vi "Temporarily Grant File Permissions.vi"(8 "error in":errorcluster) -> (0 "error out":errorcluster)   [LabVIEW 2015]
panel:
  out "permissions":i16
  out "path out":path
  in  "others":T1={"read"=TRUE, "write"=TRUE, "execute"=TRUE}
  in  "group":T1={"read"=TRUE, "write"=TRUE, "execute"=TRUE}
  in  "user":T1={"read"=TRUE, "write"=TRUE, "execute"=TRUE}
  in  "path":path=path "C:/Program Files (x86)/National Instruments/RT Images/User Components"
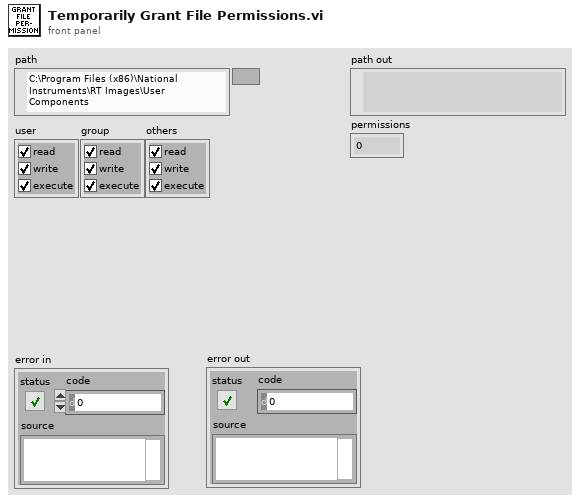
[diagram p1: front panel]
types:
  T1 = cluster{"read":bool, "write":bool, "execute":bool}
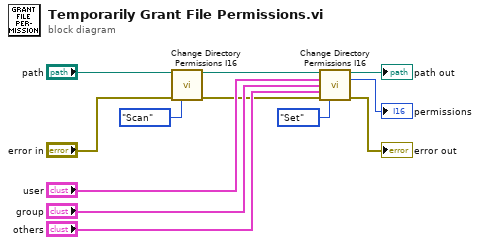
[diagram p0: block diagram]
diagram:
  n1 = call "Change Directory Permissions I16.vi"("path"="path", "error in"="error in", "Action (Get)"=enum16{"Get", "Scan", "Set", "Restore"}."Scan") -> ("path out"=w2:path, "error out"=w3:errorcluster)  [unwired: 10 in, 1 out]
  n2 = call "Change Directory Permissions I16.vi"("path"=w2, "user"="user", "group"="group", "others"="others", "error in"=w3, "Action (Get)"=enum16{"Get", "Scan", "Set", "Restore"}."Set") -> ("path out"=→"path out":path, "permissions"=→"permissions":i16, "error out"=→"error out":errorcluster)  [unwired: 7 in]
